vi "Encode UTF8toGBK.vi"(8 "error in (no error)":errorcluster, 10 "UTF-8":string="测试") -> (0 "error out":errorcluster, 2 "GBK":string)   [LabVIEW 2017, in "xHelper.lvlib"]
uses:
  xHelper.lvlib
  kernel32.dll
panel:
  out "Unicode":string
  # "\"测试\"\nUTF-8   E6B5 8BE8 AF95\nUnicode 4B6D D58B \nGBK     B2E2 CAD4"
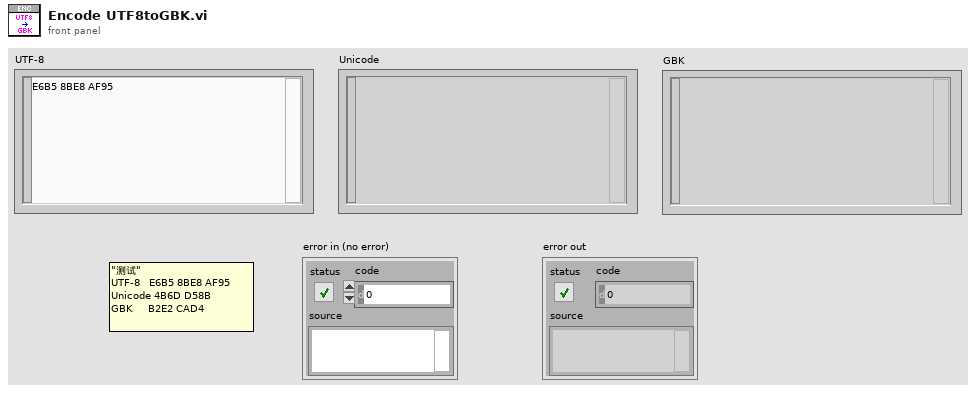
[diagram p1: front panel]
types:
  T1 = enum16{"big-endian, network order", "native, host order", "little-endian"}
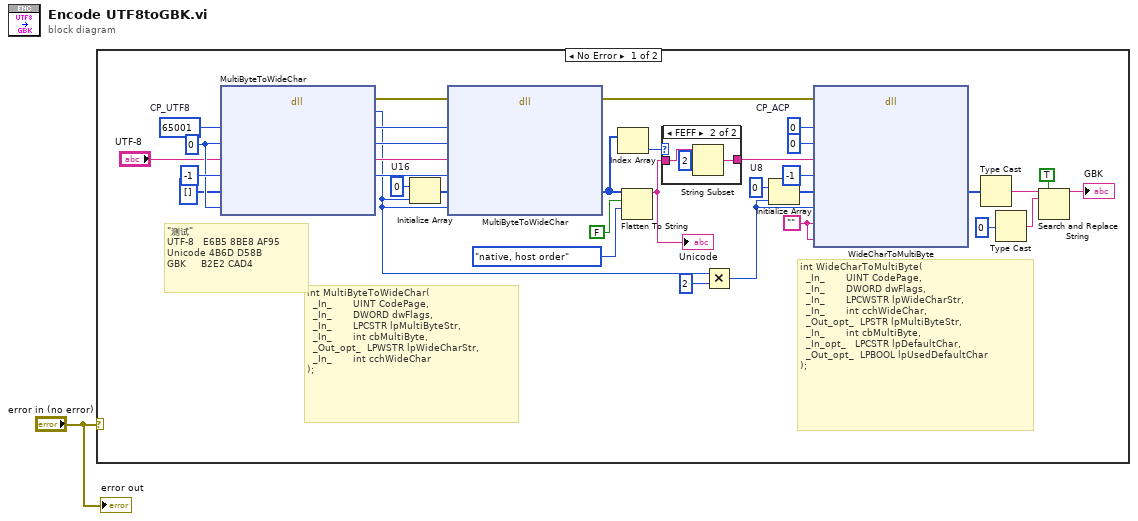
[diagram p0: block diagram]
diagram:
  n1 = case shown="No Error" "error in (no error)" {
    frame No Error {
      w20 = u8 0  # U8
      w22 = u16 0  # U16
      w16 = u32 0  # CP_ACP
      w12 = ""
      w33 = 0 ("dwFlags")
      w32 = u32 65001  # CP_UTF8
      # "int MultiByteToWideChar(\n  _In_       UINT CodePage,\n  _In_       DWORD dwFlags,\n  _In_       LPCSTR lpMultiByteStr,\n  _In_       int cbMultiByte,\n  _Out_opt_  LPWSTR lpWideCharStr,\n  _In_       int cchWideChar\n);"
      # "int WideCharToMultiByte(\n  _In_       UINT CodePage,\n  _In_       DWORD dwFlags,\n  _In_       LPCWSTR lpWideCharStr,\n  _In_       int cchWideChar,\n  _Out_opt_  LPSTR lpMultiByteStr,\n  _In_       int cbMultiByte,\n  _In_opt_   LPCSTR lpDefaultChar,\n  _Out_opt_  LPBOOL lpUsedDefaultChar\n);"
      # "\"测试\"\nUTF-8   E6B5 8BE8 AF95\nUnicode 4B6D D58B \nGBK     B2E2 CAD4"
      n2 = dll-call lib="kernel32.dll" fn="MultiByteToWideChar"("CodePage"=w32, "dwFlags"=w33, "lpMultiByteStr"="UTF-8", "cbMultiByte"=-1, "lpWideCharStr"=u16[] [], "cchWideChar"=w33) -> (error out=w35:errorcluster, "返回类型"=w9:i32, "CodePage"=w29:u32, "dwFlags"=w30:i32, "lpMultiByteStr"=w31:string, "cbMultiByte"=w28:i32)  [unwired: 5 in, 1 out]
      n3 = Initialize Array(w22, w9) -> (w21:u16[])
      n4 = dll-call lib="kernel32.dll" fn="MultiByteToWideChar"(error in=w35, "CodePage"=w29, "dwFlags"=w30, "lpMultiByteStr"=w31, "cbMultiByte"=w28, "lpWideCharStr"=w21, "cchWideChar"=w9) -> (error out=w17:errorcluster, "lpWideCharStr"=w23:u16[])  [unwired: 8 in, 1 out]
      n5 = Index Array(array=w23) -> (element=w24:u16)  [unwired: 1 in]
      n6 = Flatten To String(anything=w23, prepend array or string size? (T)=FALSE ("预置数组或字符串大小？(T)"), byte order (0:big-endian, network order)=T1."native, host order" ("字节顺序(0:big-endian, network order)")) -> (data string=w11:string)  [unwired: 1 in, 2 out]
      "Unicode" <- w11
      n7 = case shown="FEFF" w24 {
        tunnel: w11 -> [w36 w38]
        tunnel: [w36 w37] -> w14
        frame Default {
        }
        frame 65279 {
          n8 = String Subset(string=w38, offset (0)=2 ("偏移量(0)")) -> (substring=w37:string)  [unwired: 1 in]
        }
      }
      n9 = Multiply(x=w9, y=2) -> (x*y=w8:i32)
      n10 = Initialize Array(w20, w8) -> (w19:u8[])
      n11 = dll-call lib="kernel32.dll" fn="WideCharToMultiByte"(error in=w17, "CodePage"=w16, "dwFlags"=0, "lpWideCharStr"=w14, "cchWideChar"=-1, "lpMultiByteStr"=w19, "cchMultiByte"=w8, "lpDefaultChar"=w12, "pfUsedDefaultChar"=w12) -> ("lpMultiByteStr"=w7:u8[])  [unwired: 10 in, 2 out]
      n12 = Type Cast(x=w7) -> (*(type *) &x=w4:string)  [unwired: 1 in]
      n13 = Type Cast(x=u8 0 ("元素")) -> (*(type *) &x=w6:string)  [unwired: 1 in]
      n14 = Search and Replace String(replace all?=TRUE ("替换全部？(F)"), input string=w4, search string=w6) -> (result string=→"GBK":string)  [unwired: 5 in, 3 out]
    }
    frame Error {
    }
  }
  "error out" <- "error in (no error)"
